vi "DAQmx Control Relay (SubVI).vi"(0 "cDAQ Chassis":i32=1, 5 "9481 (I) Slot":i32=2, 7 "9481 (II) Slot":i32=3, 11 "Error Input":errorcluster, 12 "Relay Control":bool[](array[boolean])=[FALSE, FALSE, FALSE, FALSE, FALSE, FALSE, FALSE, FALSE], 14 "Stop Program":bool) -> (4 "Relay Task":refnum<k21>="Relay Control", 15 "Relay Error":errorcluster={"status"=TRUE, "code"=-200170, "source"="DAQmx Create Channel (DO-Digital Output).vi:1<append>\n<B>Task Name: </B>Relay Control"})   [LabVIEW 2010]
uses:
  <vilib>/DAQmx/write.llb/DAQmx Write.vi
  <vilib>/DAQmx/write.llb/DAQmx Write (Digital 1D Bool NChan 1Samp 1Line).vi
  <vilib>/DAQmx/create/channels.llb/DAQmx Create Channel (DO-Digital Output).vi
  <vilib>/daqmx/miscellaneous.llb/DAQmx Fill In Error Info.vi
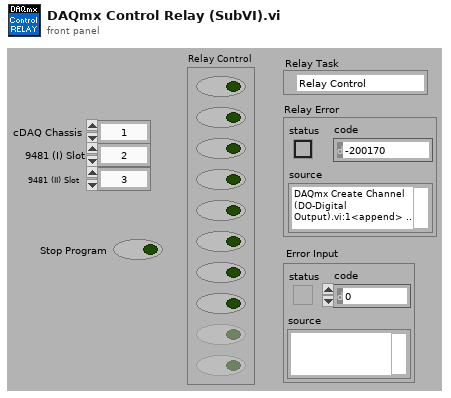
[diagram p1: front panel]
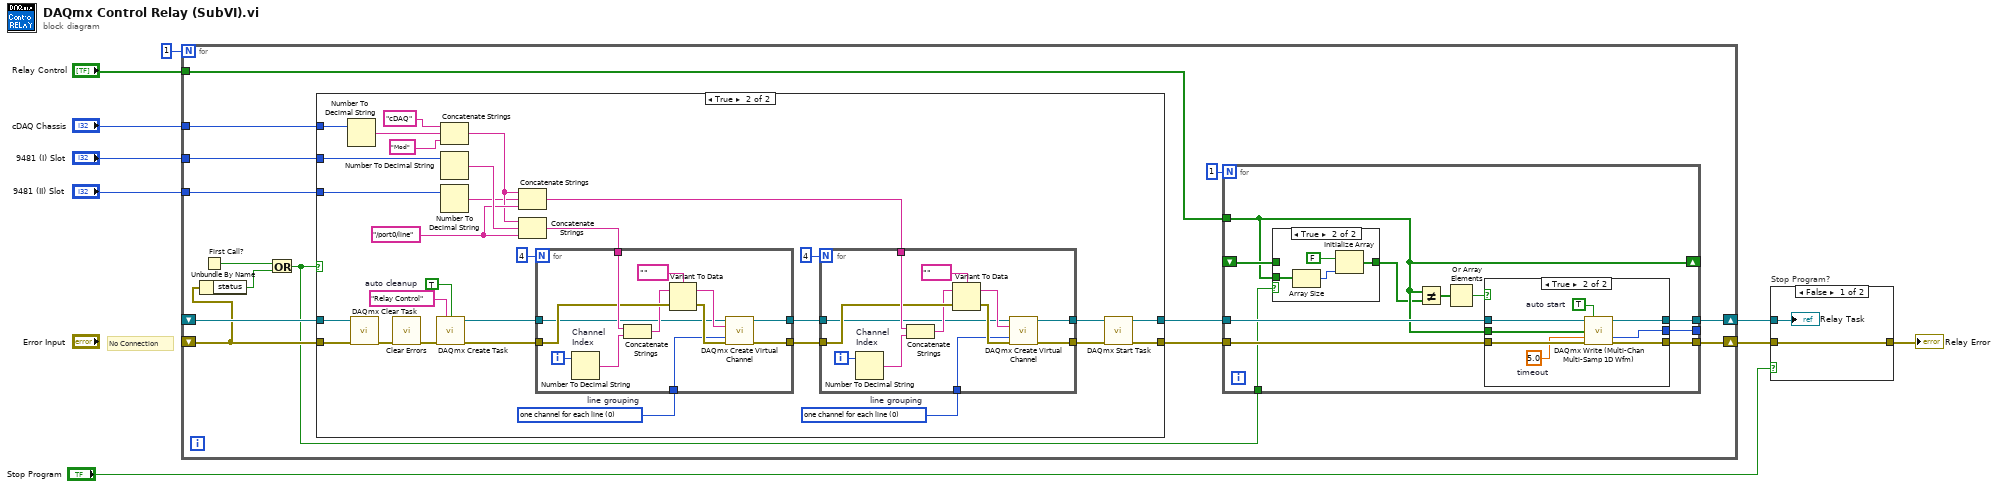
[diagram p0: block diagram]
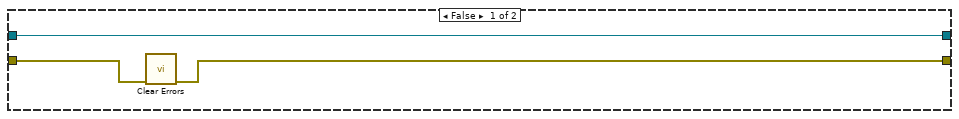
[diagram p2: hidden frame]
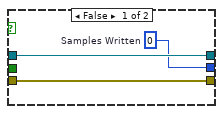
[diagram p4: hidden frame]
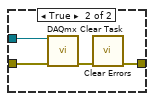
[diagram p5: hidden frame]
diagram:
  # "No Connection"
  n1 = for {
    N: 1 -> [_]
    tunnel: "9481 (I) Slot" -> [w20]
    tunnel: "cDAQ Chassis" -> [w19]
    tunnel: "9481 (II) Slot" -> [w18]
    tunnel: "Relay Control" -> [w17]
    shift-right: [w15] -> w3
    shift-left: _ -> [w14]
    shift-right: [w16] -> w4
    shift-left: _ -> [w13]
    n2 = Unbundle By Name(w13) -> ("status"=w12:bool)
    n3 = First Call?() -> (First Call?: T/F=w11:bool)
    n4 = Or(x=w11, y=w12) -> (x .or. y?=w10:bool)
    n5 = case shown="True" w10 {
      tunnel: w19 -> [_ w52]
      tunnel: w20 -> [_ w51]
      tunnel: [w26 w28] -> w22
      tunnel: [w24 w27] -> w23
      tunnel: w13 -> [w25 w43]
      tunnel: w14 -> [w26 w44]
      tunnel: w18 -> [_ w33]
      frame False {
        n6 = call <vilib>:"Clear Errors.vi"("error in (no error)"=w25) -> ("error out"=w24:errorcluster)  [unwired: 6 in]
      }
      frame True {
        w39 = 0 items=["one channel for each line", "one channel for all lines"]  # line grouping
        w48 = 0 items=["one channel for each line", "one channel for all lines"]  # line grouping
        w54 = TRUE  # auto cleanup
        w35 = "/port0/line" ("string")
        n7 = Number To Decimal String(number=w52) -> (decimal integer string=w56:string)  [unwired: 1 in]
        n8 = call <vilib>:"DAQmx Clear Task.vi"("task in"=w44, "error in"=w43) -> ("error out"=w42:errorcluster)  [unwired: 13 in]
        n9 = call <vilib>:"Clear Errors.vi"("error in (no error)"=w42) -> ("error out"=w41:errorcluster)  [unwired: 6 in]
        n10 = call <vilib>:"DAQmx Create Task.vi"("new task name"="Relay Control", "auto cleanup"=w54, "error in"=w41) -> ("task out"=w46:refnum<k21>, "error out"=w47:errorcluster)  [unwired: 11 in]
        n11 = Concatenate Strings("cDAQ" ("string"), w56, "Mod" ("string")) -> (w34:string)
        n12 = Number To Decimal String(number=w51) -> (decimal integer string=w55:string)  [unwired: 1 in]
        n13 = Number To Decimal String(number=w33) -> (decimal integer string=w32:string)  [unwired: 1 in]
        n14 = Concatenate Strings(w34, w32, w35) -> (w31:string)
        n15 = Concatenate Strings(w34, w55, w35) -> (w49:string)
        n16 = for {
          N: 4 -> [_]
          tunnel: w49 -> [w78]
          tunnel: w47 -> [w76]
          tunnel: [w70] -> w37
          tunnel: w46 -> [w72]
          tunnel: [w71] -> w38
          tunnel: w48 -> [w69]
          i -> [w79]
          n17 = Number To Decimal String "Channel\nIndex"(number=w79) -> (decimal integer string=w80:string)  [unwired: 1 in]
          n18 = Concatenate Strings(w78, w80) -> (w73:string)
          n19 = Variant To Data(error in=w76, Variant=w73, type=tag "" ("physical channels")) -> (error out=w75:errorcluster, data=w74:tag)
          n20 = call-poly <vilib>:"DAQmx Create Virtual Channel.vi"("task in"=w72, "lines"=w74, "line grouping"=w69, "error in"=w75) -> ("task out"=w71:refnum<k21>, "error out"=w70:errorcluster)  [unwired: 10 in]
        }
        n21 = for {
          N: 4 -> [_]
          tunnel: w31 -> [w66]
          tunnel: w37 -> [w64]
          tunnel: [w58] -> w29
          tunnel: w38 -> [w60]
          tunnel: [w59] -> w30
          tunnel: w39 -> [w57]
          i -> [w67]
          n22 = Number To Decimal String "Channel\nIndex"(number=w67) -> (decimal integer string=w68:string)  [unwired: 1 in]
          n23 = Concatenate Strings(w66, w68) -> (w61:string)
          n24 = Variant To Data(error in=w64, Variant=w61, type=tag "" ("physical channels")) -> (error out=w63:errorcluster, data=w62:tag)
          n25 = call-poly <vilib>:"DAQmx Create Virtual Channel.vi"("task in"=w60, "lines"=w62, "line grouping"=w57, "error in"=w63) -> ("task out"=w59:refnum<k21>, "error out"=w58:errorcluster)  [unwired: 10 in]
        }
        n26 = call <vilib>:"DAQmx Start Task.vi"("task/channels in"=w30, "error in"=w29) -> ("task out"=w28:refnum<k21>, "error out"=w27:errorcluster)  [unwired: 12 in]
      }
    }
    n27 = for {
      N: 1 -> [_]
      tunnel: w22 -> [w91]
      tunnel: w23 -> [w90]
      tunnel: w17 -> [w82]
      shift-right: [w82] -> _
      shift-left: _ -> [w83]
      tunnel: [w89] -> w16
      tunnel: [w88] -> _
      tunnel: [w87] -> w15
      tunnel: w10 -> [w84]
      n28 = case shown="True" w84 {
        tunnel: w82 -> [_ w94]
        tunnel: [w92 w93] -> w81
        tunnel: w83 -> [w92 _]
        frame False {
        }
        frame True {
          n29 = Array Size(array=w94) -> (size(s)=w95:i32)
          n30 = Initialize Array(FALSE, w95) -> (w93:bool[])
        }
      }
      n31 = Not Equal?(x=w82, y=w81) -> (x != y?=w86:bool[])
      n32 = Or Array Elements(Boolean array=w86) -> (logical OR=w85:bool)
      n33 = case shown="True" w85 {
        tunnel: w91 -> [w99 w106]
        tunnel: w90 -> [w97 w105]
        tunnel: w82 -> [_ w104]
        tunnel: [w97 w103] -> w89
        tunnel: [w98 w101] -> w88
        tunnel: [w99 w100] -> w87
        frame False {
          w98 = u32 0  # Samples Written
        }
        frame True {
          w102 = 5.0  # timeout
          w107 = TRUE  # auto start
          n34 = call-poly "DAQmx Write (Multi-Chan Multi-Samp 1D Wfm).vi"("task/channels in"=w106, "auto start"=w107, "data"=w104, "timeout"=w102, "error in"=w105) -> ("task out"=w100:refnum<k21>, "number of samples written per channel"=w101:u32, "error out"=w103:errorcluster)  [unwired: 8 in]
        }
      }
    }
  }
  n35 = case "Stop Program?" shown="False" "Stop Program" {
    tunnel: w3 -> [w109 w111]
    tunnel: w4 -> [w108 w112]
    tunnel: [w108 w110] -> w5
    frame False {
      "Relay Task" <- w109
    }
    frame True {
      n36 = call <vilib>:"DAQmx Clear Task.vi"("task in"=w111, "error in"=w112) -> ("error out"=w113:errorcluster)  [unwired: 13 in]
      n37 = call <vilib>:"Clear Errors.vi"("error in (no error)"=w113) -> ("error out"=w110:errorcluster)  [unwired: 6 in]
    }
  }
  "Relay Error" <- w5
